vi "Read.vi"(8 "error in (no error)":errorcluster, 11 "String in":refnum<class "Const_Str_1D.lvclass">) -> (0 "error out":errorcluster, 2 "Array":string[](array[string]), 3 "String out":refnum<class "Const_Str_1D.lvclass">)   [LabVIEW 2021, in "Const_Str_1D.lvclass"]
uses:
  Const_Str_1D.lvclass
  Const_Str_1D.lvclass/Const_Str_1D.ctl
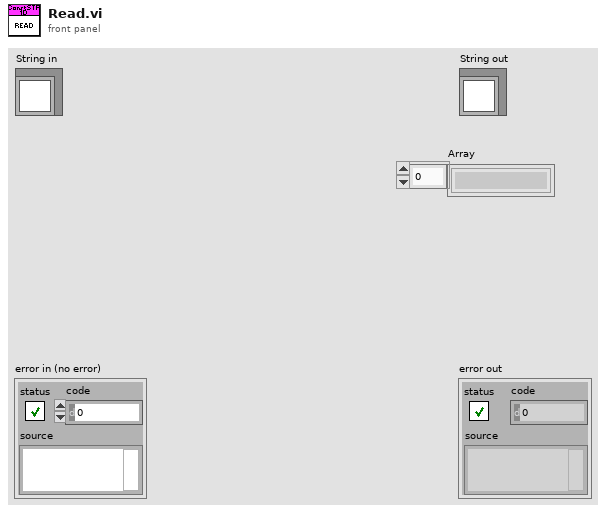
[diagram p1: front panel]
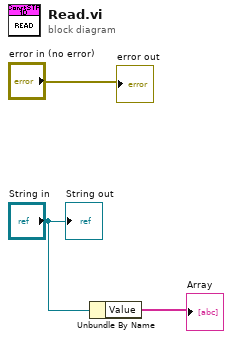
[diagram p0: block diagram]
diagram:
  n1 = Unbundle By Name("String in") -> ("Value"=→"Array":string[])
  "error out" <- "error in (no error)"
  "String out" <- "String in"
